vi "FestoCPX.Station.Emg.Check.vi"(8 "error in":errorcluster) -> (0 "error out":errorcluster, 1 "Emg occured":bool, 2 "Emg":T1)   [LabVIEW 2016]
uses:
  FestoCPX.Station.EmgState.ctl
  FestoCPX.DI.Signal.ctl
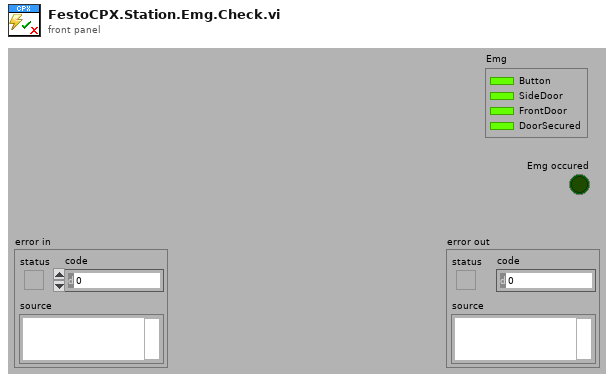
[diagram p1: front panel]
types:
  T1 = typedef "FestoCPX.Station.EmgState.ctl" = cluster{"Button":bool, "SideDoor":bool, "FrontDoor":bool, "DoorSecured":bool}
  T2 = typedef "FestoCPX.DI.Signal.ctl" = enum16{"S.C. Emergency Stop", "S.C. Side Door Close", "S.C. Front Door Close", "S.C. Front Door Secured", "Button Start", "Button Stop", "Button Control", "Product Move Home", "Product Move Work", "Table Position", "Table Lock", "Product Lift A Home", "Product Lift B Home", "Product Arm OK", "Product Arm NOK", "Product Arm Work", "Revolver ID 1", "Revolver ID 2", "Revolver ID 3", "Revolver ID 4", "Revolver ID 5", "Air Pressure Inside", "Air Pressure Inlet", "Product Slot 1 A Present", "Product Slot 1 B Present", "Product Slot 2 A Present", "Product Slot 2 B Present", "Product Slot 3 A Present", "Product Slot 3 B Present", "Product Slot 4 A Present", "Product Slot 4 B Present", "Product Final A Present", "Product Final B Present", "Product Output A Present", "Product Output B Present", "Product Container OK Present", "Product Container NOK Present", "Fork ID 1", "Fork ID 2"}
  T3 = cluster{"[0]":bool, "[1]":bool, "[2]":bool, "[3]":bool}
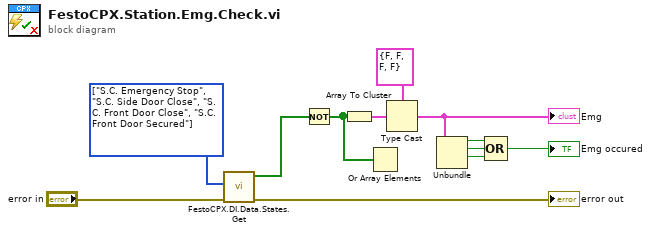
[diagram p0: block diagram]
diagram:
  w9 = T2[] [enum."S.C. Emergency Stop", enum."S.C. Side Door Close", enum."S.C. Front Door Close", enum."S.C. Front Door Secured"] items=["S.C. Emergency Stop", "S.C. Side Door Close", "S.C. Front Door Close", "S.C. Front Door Secured", "Button Start", "Button Stop", "Button Control", "Product Move Home", "Product Move Work", "Table Position", "Table Lock", "Product Lift A Home", "Product Lift B Home", "Product Arm OK", "Product Arm NOK", "Product Arm Work", "Revolver ID 1", "Revolver ID 2", "Revolver ID 3", "Revolver ID 4", "Revolver ID 5", "Air Pressure Inside", "Air Pressure Inlet", "Product Slot 1 A Present", "Product Slot 1 B Present", "Product Slot 2 A Present", "Product Slot 2 B Present", "Product Slot 3 A Present", "Product Slot 3 B Present", "Product Slot 4 A Present", "Product Slot 4 B Present", "Product Final A Present", "Product Final B Present", "Product Output A Present", "Product Output B Present", "Product Container OK Present", "Product Container NOK Present", "Fork ID 1", "Fork ID 2"] ("CPX.DI")
  n1 = call "FestoCPX.DI.Data.States.Get.vi"("error in (no error)"="error in", "CPX.DI"=w9) -> ("error out"=→"error out":errorcluster, "State"=w1:bool[])  [unwired: 5 in, 3 out]
  n2 = Not(x=w1) -> (.not. x?=w7:bool[])
  n3 = Array To Cluster(array=w7) -> (cluster=w11:T3)
  n4 = Or Array Elements(Boolean array=w7) -> ()  [unwired: 1 out]
  n5 = Type Cast(type=T1 {"Button"=FALSE, "SideDoor"=FALSE, "FrontDoor"=FALSE, "DoorSecured"=FALSE} ("Emg"), x=w11) -> (*(type *) &x=w6:T1)
  "Emg" <- w6
  n6 = Unbundle(w6) -> ("Button"=w5:bool, "SideDoor"=w4:bool, "FrontDoor"=w3:bool)  [unwired: 1 out]
  n7 = Compound Arithmetic op=OR(w5, w4, w3) -> (→"Emg occured":bool)
